vi "AcquireData.vi"(8 "error in (no error)":errorcluster, 11 "DAQ in":refnum<class "DAQ.lvclass">) -> (0 "error out":errorcluster, 3 "DAQ out":refnum<class "DAQ.lvclass">)   [LabVIEW 2011, in "DAQ.lvclass"]
uses:
  DAQ.lvclass
  Messages/Data Update Msg/Data Update Msg.lvclass
  Controls/Extended Arduino Commands.ctl
  <userlib>/_Frameworks/ActorFramework/Actor/Actor.lvclass/Actor.ctl
  DAQ.lvclass/DAQ.ctl
  <vilib>/LabVIEW Interface for Arduino/LabVIEW Interface for Arduino.lvlib
  <userlib>/_Frameworks/ActorFramework/Actor/Actor.lvclass
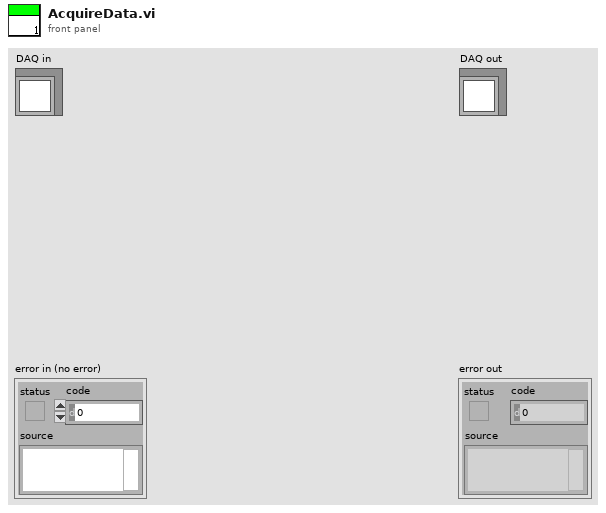
[diagram p1: front panel]
types:
  T1 = typedef "DAQ.lvclass/Extended Arduino Commands.ctl" = u8
  T2 = typedef "LabVIEW Interface for Arduino.lvlib/Arduino Resource.ctl" = cluster{"VISA resource":refnum<visa-resource-name>, "Board Type":T3, "Connection Type":enum8{"USB / Serial"}, "Bytes Per Packet (15)":u8}
  T3 = typedef "LabVIEW Interface for Arduino.lvlib/Board Type.ctl" = enum16{"Uno", "Dimuelanove w/Atmega 328", "Mega 2560"}
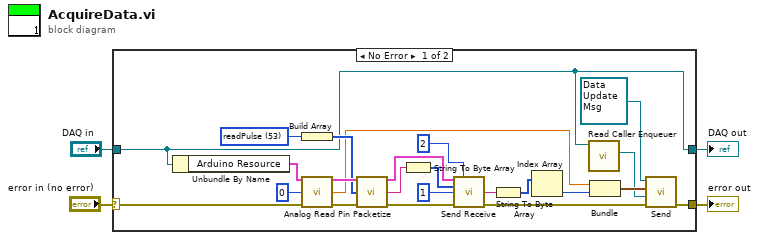
[diagram p0: block diagram]
diagram:
  n1 = case shown="No Error" "error in (no error)" {
    selector: "error in (no error)" -> [w16 w29]
    tunnel: [w6 w29] -> w3
    tunnel: [w9 w28] -> w1
    tunnel: "DAQ in" -> [w9 w28]
    frame No Error {
      w23 = T1 53 items=["readPulse"=53] ("Menu Ring")
      n2 = Unbundle By Name(w9) -> ("Arduino Resource"=w27:T2)
      n3 = Build Array(w23) -> (w24:T1[])
      n4 = call <vilib>:"Analog Read Pin.vi"("Arduino Resource"=w27, "Analog Input Pin (0)"=u8 0, "error in"=w16) -> ("Arduino Resource"=w26:T2, "Voltage"=w11:dbl, "error out"=w25:errorcluster)  [unwired: 10 in]
      n5 = call <vilib>:"Packetize.vi"("Arduino Resource"=w26, "Data"=w24, "error in"=w25) -> ("Arduino Resource"=w22:T2, "Packet"=w20:string, "error out"=w21:errorcluster)  [unwired: 10 in]
      n6 = String To Byte Array(string=w20) -> (unsigned byte array=w19:u8[])
      n7 = call <vilib>:"Send Receive.vi"("Arduino Resource"=w22, "Max Retries  (10)"=2, "Data"=w19, "Bytes To Read (0)"=u8 1, "error in"=w21) -> ("Read Buffer"=w14:string, "error out"=w7:errorcluster)  [unwired: 8 in, 1 out]
      n8 = String To Byte Array(string=w14) -> (unsigned byte array=w13:u8[])
      n9 = Index Array(array=w13) -> (element=w12:u8)  [unwired: 1 in]
      n10 = call <userlib>:"Read Caller Enqueuer.vi"("Actor"=w9) -> ("Caller Enqueuer"=w8:refnum<class "Message Enqueuer.lvclass">)  [unwired: 10 in]
      n11 = Bundle("Voltage"=w11, w12) -> (w10:cluster{"Voltage":dbl, u8})  [unwired: 1 in]
      n12 = call "Send.vi"("error in (no error)"=w7, "Queue"=w8, "Data"=w10, "Data Update Msg in"=refnum<class "Data Update Msg.lvclass"> refnum) -> ("error out"=w6:errorcluster)  [unwired: 6 in, 1 out]
    }
    frame Error {
    }
  }
  "error out" <- w3
  "DAQ out" <- w1
